vi "Send Embedded Progress Bar Update.vi"(6 "Stop Progress Bar (F)":bool, 8 "Error In":errorcluster, 9 "Max Iterations N":i32, 10 "Current Iteration i (i or -1: standard or || iteration; 0 or -2: first standard or || iteration)":i32=-1, 11 "Progress Bar Queue in":refnum<queue>) -> (0 "Error Out":errorcluster, 3 "Progress Bar Queue out":refnum<queue>)   [LabVIEW 2021, in "GUI.lvlib"]
doc: "Pass -2 before the first iteration for <b>Current Iteration i</b> and -1 on subsequent iterations. The <b>Max Iterations N</b> parameter is only needed on the first iteration and should be passed outside the loop with the value -2 for i.\n\nWire True to <b>Stop Progress Bar</b> to hide the Progress Bar (usually done outside a loop after completion of the task requiring the progress bar)."
uses:
  GUI.lvlib
  Embedded Progress Bar Q Element.ctl
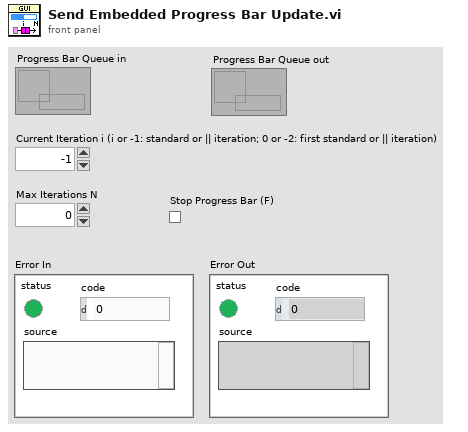
[diagram p1: front panel]
types:
  T1 = typedef "GUI.lvlib/Embedded Progress Bar Q Element.ctl" = cluster{"Action":string, "Value":dbl}
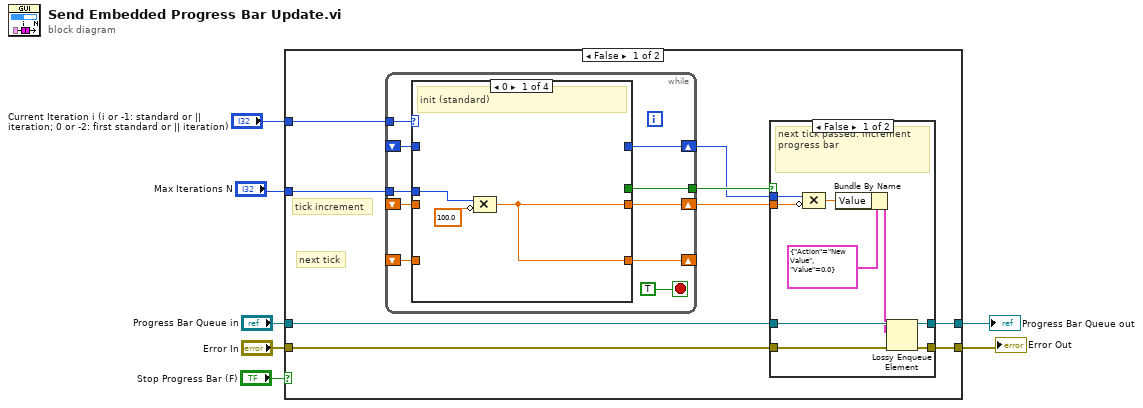
[diagram p0: block diagram]
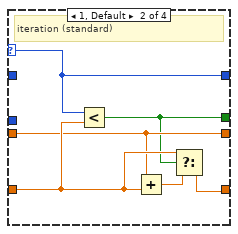
[diagram p2: hidden frame]
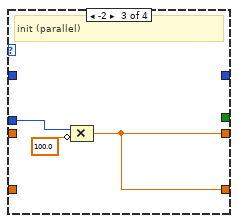
[diagram p3: hidden frame]
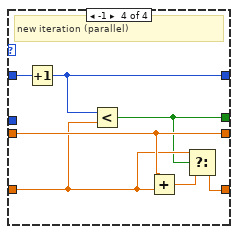
[diagram p4: hidden frame]
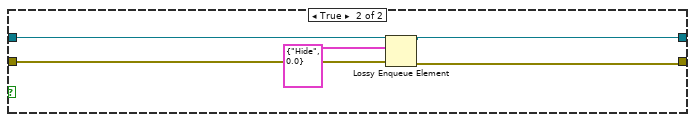
[diagram p6: hidden frame]
diagram:
  n1 = case shown="False" "Stop Progress Bar (F)" {
    tunnel: "Progress Bar Queue in" -> [w16 w61]
    tunnel: "Current Iteration i (i or -1: standard or || iteration; 0 or -2: first standard or || iteration)" -> [w12 _]
    tunnel: "Error In" -> [w15 w60]
    tunnel: [w14 w58] -> w4
    tunnel: [w13 w57] -> w3
    tunnel: "Max Iterations N" -> [w11 _]
    frame False {
      # "tick increment"
      # "next tick"
      n2 = while {
        tunnel: w12 -> [w26]
        shift-right: [w25] -> w9
        shift-left: _ -> [w24]
        tunnel: w11 -> [w23]
        shift-right: [w22] -> w8
        shift-left: _ -> [w21]
        shift-right: [w19] -> _
        shift-left: _ -> [w18]
        tunnel: [w17] -> w10
        stop <- TRUE stop-if-true
        n3 = case shown="0" w26 {
          selector: w26 -> [_ w35 _ _]
          tunnel: [_ w35 _ w43] -> w25
          tunnel: w24 -> [_ _ _ w45]
          tunnel: w23 -> [w29 _ w38 _]
          tunnel: [w27 w33 w36 w42] -> w22
          tunnel: w21 -> [_ w33 _ w42]
          tunnel: [w27 w32 w36 w39] -> w19
          tunnel: w18 -> [_ w34 _ w41]
          tunnel: [_ w30 _ w40] -> w17
          frame 0 {
            # "init (standard)"
            n4 = Compound Arithmetic op=MULTIPLY(w29, invert 100.0 ("y")) -> (w27:dbl)
          }
          frame 1, Default {
            # "iteration (standard)"
            n5 = Less?(x=w35, y=w34) -> (x < y?=w30:bool)
            n6 = Add(x=w33, y=w34) -> (x+y=w31:dbl)
            n7 = Select(t=w34, s=w30, f=w31) -> (s? t:f=w32:dbl)
          }
          frame -2 {
            # "init (parallel)"
            n8 = Compound Arithmetic op=MULTIPLY(w38, invert 100.0 ("y")) -> (w36:dbl)
          }
          frame -1 {
            # "new iteration (parallel)"
            n9 = Increment(x=w45) -> (x+1=w43:i32)
            n10 = Less?(x=w43, y=w41) -> (x < y?=w40:bool)
            n11 = Add(x=w42, y=w41) -> (x+y=w44:dbl)
            n12 = Select(t=w41, s=w40, f=w44) -> (s? t:f=w39:dbl)
          }
        }
      }
      n13 = case shown="False" w10 {
        tunnel: w16 -> [w54 w55]
        tunnel: w15 -> [w51 w56]
        tunnel: [w50 w56] -> w14
        tunnel: [w49 w55] -> w13
        tunnel: w9 -> [w48 _]
        tunnel: w8 -> [w46 _]
        frame False {
          # "next tick passed: increment progress bar"
          n14 = Compound Arithmetic op=MULTIPLY(w48, invert w46) -> (w47:dbl)
          n15 = Bundle By Name(cluster=T1 {"Action"="New Value", "Value"=0.0} ("element"), "Value"=w47) -> (w52:T1)
          n16 = Lossy Enqueue Element(queue=w54, element=w52, error in (no error)=w51) -> (queue out=w49:refnum<queue>, error out=w50:errorcluster)  [unwired: 2 out]
        }
        frame True {
          # "next tick not reached:\ndo nothing"
        }
      }
    }
    frame True {
      n17 = Lossy Enqueue Element(queue=w61, element=T1 {"Action"="Hide", "Value"=0.0}, error in (no error)=w60) -> (queue out=w57:refnum<queue>, error out=w58:errorcluster)  [unwired: 2 out]
    }
  }
  "Error Out" <- w4
  "Progress Bar Queue out" <- w3
